vi "MT_generate_signal4.vi"(7 "Direction":bool, 8 "error in (no error)":errorcluster, 9 "# cycles":dbl, 10 "frequency":dbl, 11 "amplitude":dbl) -> (0 "error out":errorcluster, 2 "signals out":dbl[][](array[numeric]), 3 "# samples":dbl)   [LabVIEW 2019]
uses:
  <vilib>/Analysis/NI_AALBase.lvlib
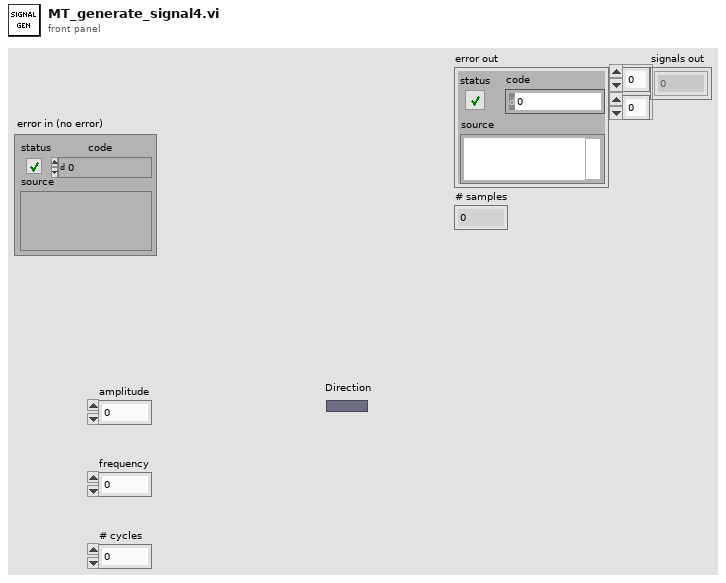
[diagram p1: front panel]
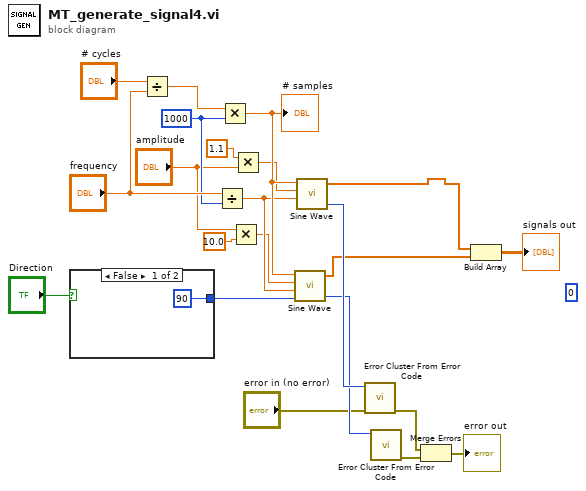
[diagram p0: block diagram]
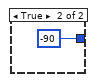
[diagram p2: hidden frame]
diagram:
  (unwired) 0 ("index")
  w19 = 1000
  n1 = case shown="False" "Direction" {
    tunnel: [90 -90] -> w5
    frame False {
    }
    frame True {
    }
  }
  n2 = Divide(x="# cycles", y="frequency") -> (x/y=w20:dbl)
  n3 = Divide(x="frequency", y=w19) -> (x/y=w17:dbl)
  n4 = Multiply(x=w20, y=w19) -> (x*y=w18:dbl)
  "# samples" <- w18
  n5 = Multiply(x="amplitude", y=10.0) -> (x*y=w15:dbl)
  n6 = Multiply(x=1.1, y="amplitude") -> (x*y=w6:dbl)
  n7 = call <vilib>:"Sine Wave.vi"("samples"=w18, "amplitude"=w15, "frequency"=w17, "phase in"=w5) -> ("sine wave"=w1:dbl[], "error"=w13:i32)  [unwired: 1 in, 1 out]
  n8 = call <vilib>:"Sine Wave.vi"("samples"=w18, "amplitude"=w6, "frequency"=w17) -> ("sine wave"=w2:dbl[], "error"=w14:i32)  [unwired: 2 in, 1 out]
  n9 = call <vilib>:"Error Cluster From Error Code.vi"("error in (no error)"="error in (no error)", "error code (0)"=w14) -> ("error out"=w11:errorcluster)  [unwired: 7 in]
  n10 = call <vilib>:"Error Cluster From Error Code.vi"("error code (0)"=w13) -> ("error out"=w10:errorcluster)  [unwired: 8 in]
  n11 = Merge Errors(w11, w10) -> (→"error out":errorcluster)
  n12 = Build Array(w2, w1) -> (→"signals out":dbl[][])
